vi "CreateChart.vi"(0 "reference in":refnum<class "LcWebView.lvclass">, 1 "Chart Setup":T1, 5 "error in (no error)":errorcluster) -> (14 "reference out":refnum<class "LcWebView.lvclass">, 19 "error out":errorcluster)   [LabVIEW 2018, in "LcWebView.lvclass"]
uses:
  LcWebView.lvclass
  ctrls/ChartSetup.ctl
  ctrls/ChartContent.ctl
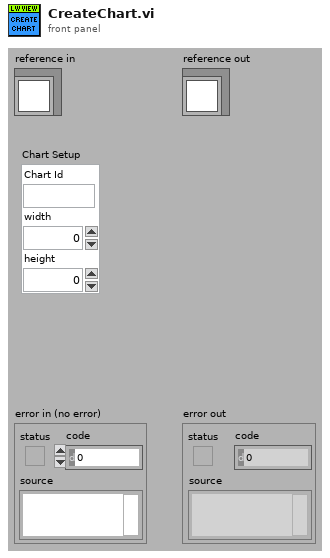
[diagram p1: front panel]
types:
  T1 = typedef "LcWebView.lvclass/ChartSetup.ctl" = cluster{"Chart Id":string, "width":u32, "height":u32}
  T2 = typedef "LcWebView.lvclass/ChartContent.ctl" = cluster{"Chart Id":string, "Chart Setup":T1, "Chart HTML":string, "Chart Config":string, "Chart Data":string}
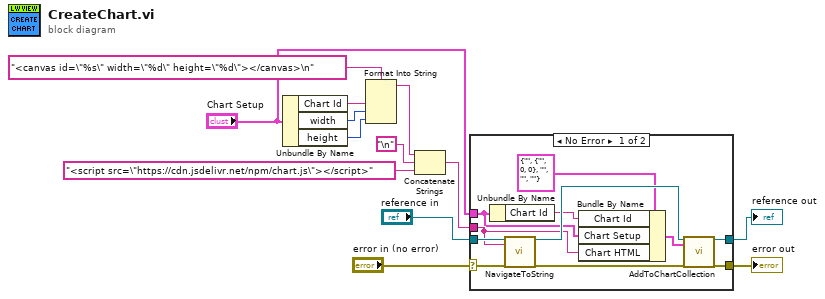
[diagram p0: block diagram]
diagram:
  n1 = Unbundle By Name("Chart Setup") -> ("Chart Id"=w2:string, "width"=w4:u32, "height"=w3:u32)
  n2 = Format Into String(format string="<canvas id=\"%s\" width=\"%d\" height=\"%d\"></canvas>\n" ("HTML Content"), w2, w4, w3) -> (resulting string=w6:string)  [unwired: 2 in, 1 out]
  n3 = Concatenate Strings(w6, "\n", "<script src=\"https://cdn.jsdelivr.net/npm/chart.js\"></script>" ("string")) -> (w5:string)
  n4 = case shown="No Error" "error in (no error)" {
    selector: "error in (no error)" -> [w24 w26]
    tunnel: [w20 w26] -> w12
    tunnel: [w21 w25] -> w10
    tunnel: "reference in" -> [w23 w25]
    tunnel: w5 -> [w18 _]
    tunnel: "Chart Setup" -> [w17 _]
    frame No Error {
      n5 = Unbundle By Name(w17) -> ("Chart Id"=w16:string)
      n6 = call-dynamic "NavigateToString.vi"("reference in"=w23, "HTML Content"=w18, "Error In"=w24) -> ("reference out"=w22:refnum<class "LcWebView.lvclass">, "Error Out"=w19:errorcluster)  [unwired: 14 in, 1 out]
      n7 = Bundle By Name(cluster=T2 {"Chart Id"="", "Chart Setup"={"Chart Id"="", "width"=0, "height"=0}, "Chart HTML"="", "Chart Config"="", "Chart Data"=""} ("Chart Content"), "Chart Id"=w16, "Chart Setup"=w17, "Chart HTML"=w18) -> (w14:T2)
      n8 = call-dynamic "AddToChartCollection.vi"("reference in"=w22, "Chart Content"=w14, "error in (no error)"=w19) -> ("reference out"=w21:refnum<class "LcWebView.lvclass">, "error out"=w20:errorcluster)  [unwired: 15 in]
    }
    frame Error {
    }
  }
  "error out" <- w12
  "reference out" <- w10
